vi "Generate Simulated Data.vi"(8 "error in (no error)":errorcluster, 9 "Hardware Resources in":T1) -> (0 "error out":errorcluster, 2 "Graph Data":waveform(dbl)[](array[waveform]))   [LabVIEW 2016, in "Acquisition.lvlib"]
doc: "Generates sample waveforms according to the signal type in the HW Config input."
uses:
  Acquisition.lvlib
  Hardware Configuration.ctl
  <vilib>/NI Modbus.llb/MB Serial Master Query Read Input Registers (poly).vi
  Global.vi
panel:
  out "Input Registers":u16[](array[numeric])
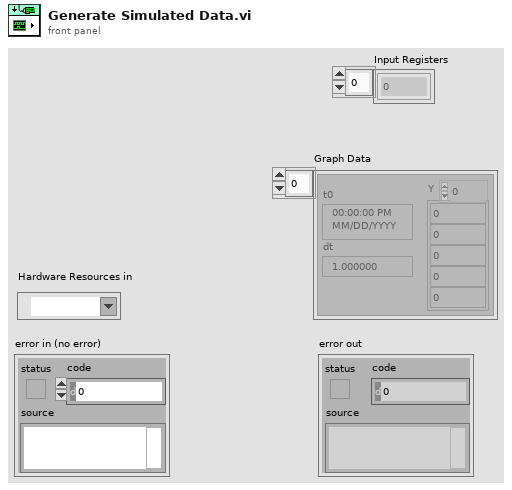
[diagram p1: front panel]
types:
  T1 = typedef "Acquisition.lvlib/Hardware Configuration.ctl" = refnum<visa-resource-name>
  T2 = cluster{"Mode":enum16{"RTU", "ASCII"}, "Slave Address":u8}
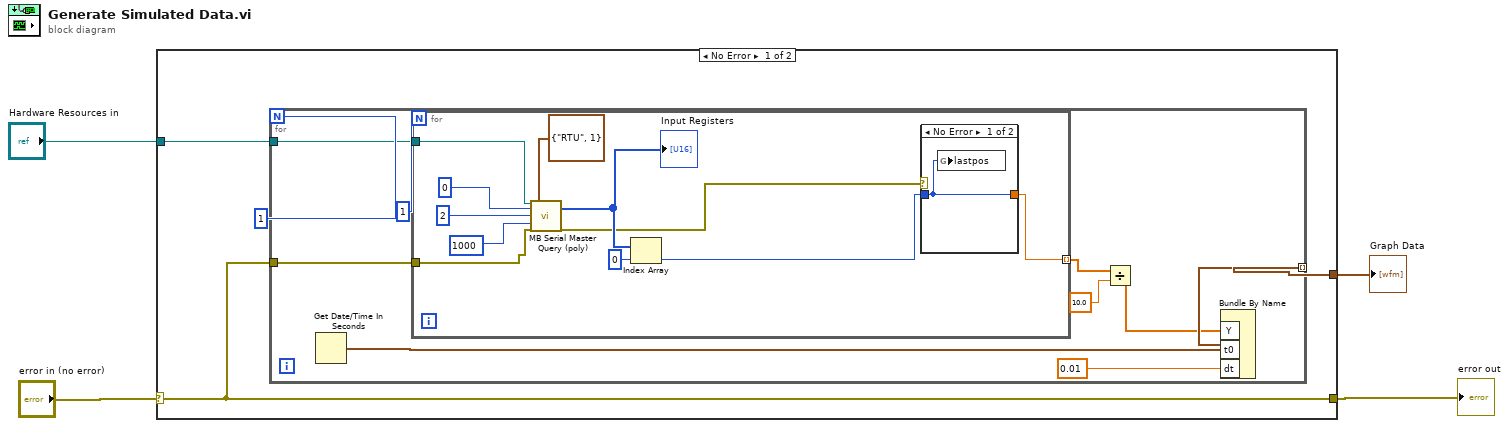
[diagram p0: block diagram]
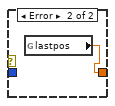
[diagram p2: hidden frame]
diagram:
  n1 = case shown="No Error" "error in (no error)" {
    selector: "error in (no error)" -> [w5 w31]
    tunnel: [w5 w31] -> w1
    tunnel: [w8 _] -> w3
    tunnel: "Hardware Resources in" -> [w6 _]
    frame No Error {
      n2 = for {
        N: 1 -> [_]
        tunnel: [w14] -> w8 mode=indexing
        tunnel: w6 -> [w12]
        tunnel: w5 -> [w11]
        n3 = Get Date/Time In Seconds() -> (seconds since 1Jan1904=w15:timestamp)
        n4 = for {
          N: 1 -> [_]
          tunnel: w12 -> [w28]
          tunnel: w11 -> [w24]
          tunnel: [w18] -> w10 mode=indexing
          n5 = call-poly <vilib>:"MB Serial Master Query (poly).vi"("VISA resource name"=w28, "Starting Address"=u16 0, "Quantity"=u16 2, "Timeout"=u32 1000, "error in"=w24, "Serial Parameters"=T2 {"Mode"=enum."RTU", "Slave Address"=1}) -> ("Input Registers"=w23:u16[], "error out"=w20:errorcluster)  [unwired: 10 in, 2 out]
          "Input Registers" <- w23
          n6 = Index Array(array=w23, index=0) -> (element=w19:u16)
          n7 = case shown="No Error" w20 {
            tunnel: [w29 w30] -> w18
            tunnel: w19 -> [w29 _]
            frame No Error {
              n8 = global write "Global.vi" "lastpos"(w29) -> ()
            }
            frame Error {
              n9 = global read "Global.vi" "lastpos"() -> (w30:dbl)
            }
          }
        }
        n10 = Divide(x=w10, y=10.0) -> (x/y=w13:dbl[])
        n11 = Bundle By Name("Y"=w13, "t0"=w15, "dt"=0.01) -> (w14:waveform(dbl))  [unwired: 1 in]
      }
    }
    frame Error {
    }
  }
  "error out" <- w1
  "Graph Data" <- w3
